vi "main.vi"() -> ()   [LabVIEW 2023]
uses:
  VoltageDataAquisition/VoltageDataAquisition.lvlib
panel:
  in  "Select Module":i32(ring)=-1 caption="Select Module\nTo send Request to" items=["All"=-1]
  in  "List":i32[](listbox)
  in  "delete":bool
  in  "add":bool
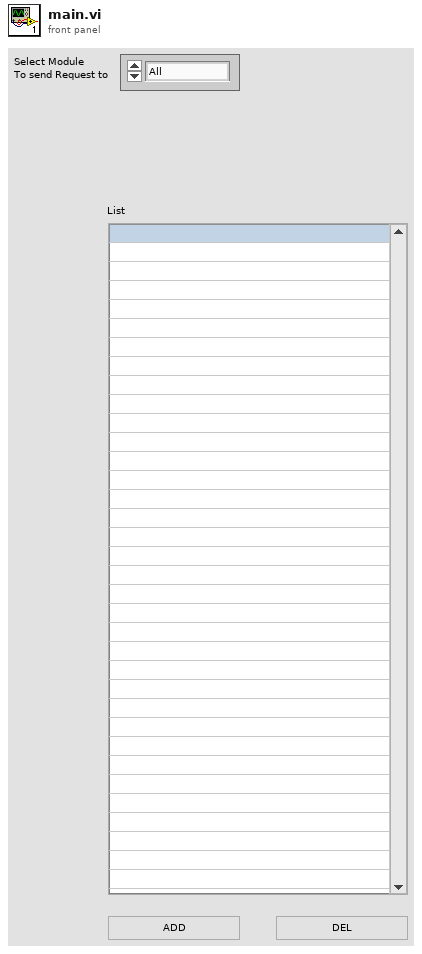
[diagram p1: front panel]
types:
  T1 = typedef "VoltageDataAquisition.lvlib/Broadcast Events--cluster.ctl" = cluster{"Module Did Init":refnum<user-event>, "Status Updated":refnum<user-event>, "Error Reported":refnum<user-event>, "Module Did Stop":refnum<user-event>, "Update Module Execution Status":refnum<user-event>}
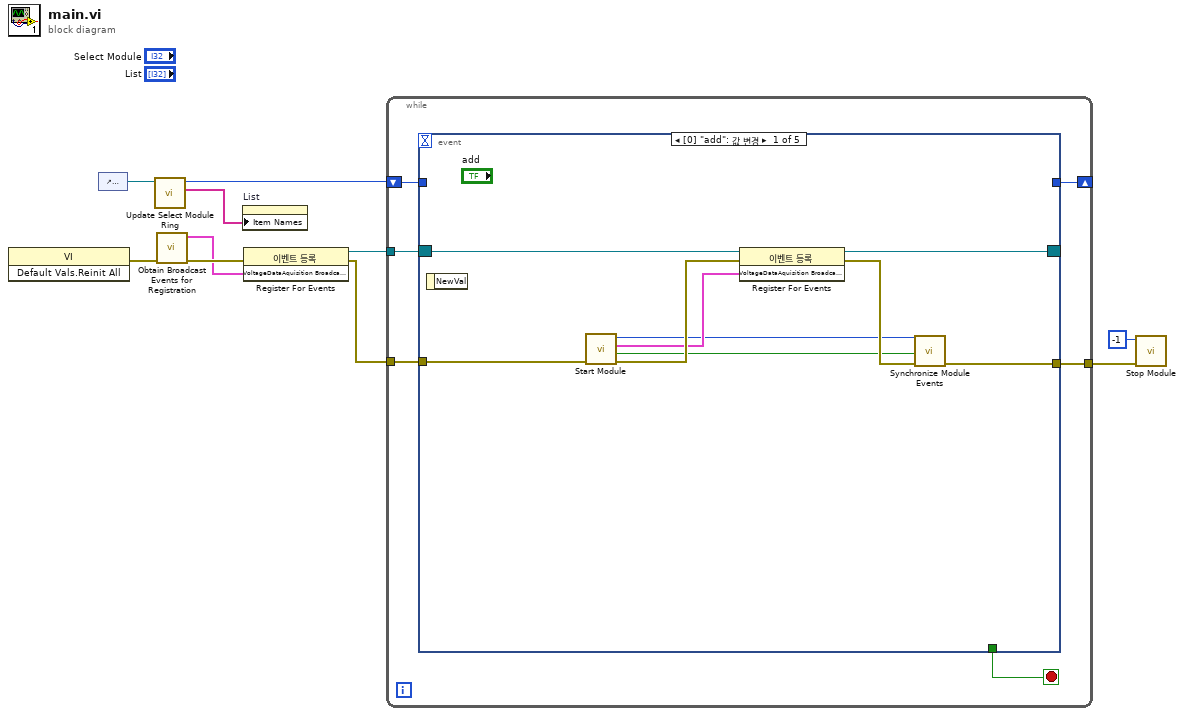
[diagram p0: block diagram]
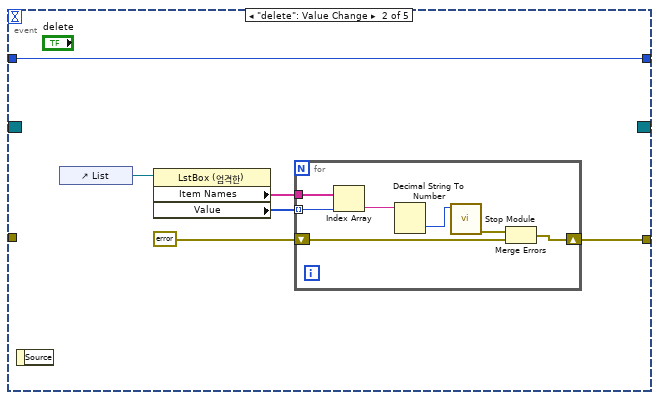
[diagram p2: hidden frame]
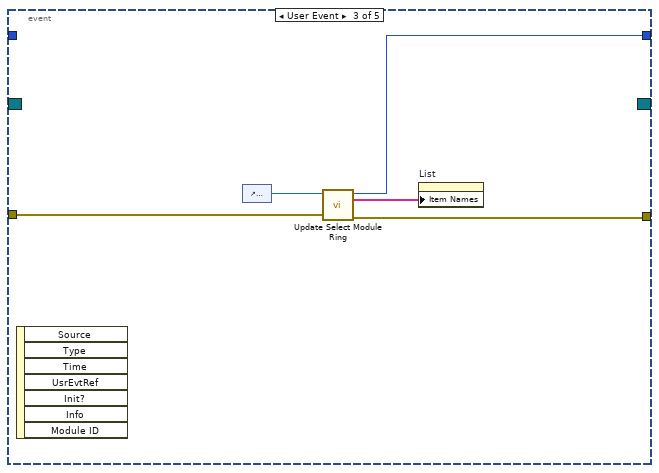
[diagram p3: hidden frame]
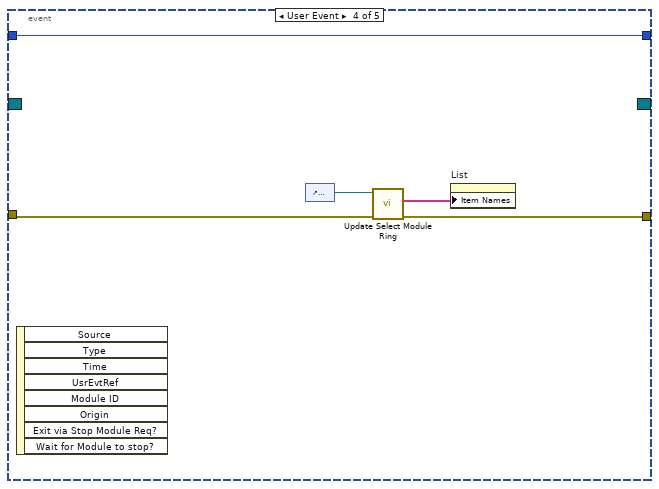
[diagram p4: hidden frame]
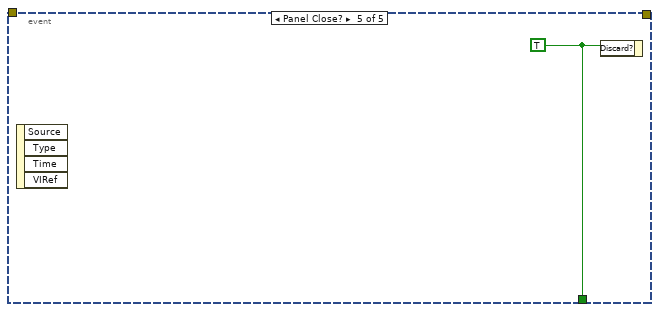
[diagram p5: hidden frame]
diagram:
  n1 = invoke class="VI" method="Default Vals.Reinit All"() -> (error out=w10:errorcluster)  [unwired: 3 in, 2 out]
  n2 = control-ref of="Select Module"() -> (w3:refnum<vi>)
  n3 = call "Update Select Module Ring.vi"("Select Module Ring Ref"=w3) -> ("Active Modules (Array)"=w1:string[], "New Module Ring Value"=w2:i32)  [unwired: 8 in, 1 out]
  n4 = call "Obtain Broadcast Events for Registration.vi"("error in"=w10) -> ("error out"=w9:errorcluster, "VoltageDataAquisition Broadcast Events"=w8:T1)  [unwired: 8 in, 1 out]
  n5 = property on="List" class="LstBox (엄격한)"("Item Names"=w1) -> ()  [unwired: 2 in, 2 out]
  n6 = register-events(error in=w9, w8) -> (reference out=w7:refnum<event-registration>, error out=w6:errorcluster)  [unwired: 1 in]
  n7 = while {
    tunnel: w7 -> [w16]
    tunnel: w6 -> [w15]
    tunnel: [w13] -> w4
    shift-right: [w11] -> _
    shift-left: w2 -> [w12]
    stop <- w14 stop-if-true
    n8 = event shown="[0] \"add\": 값 변경" {
      selector: w16 -> [w23 _ _ _ _]
      dyn-events: [w20 _ _ _ _] -> _
      timeout: _ -> [_ _ _ _ _]
      tunnel: w15 -> [w22 _ w43 w45 _]
      tunnel: [w18 w28 w42 w48 _] -> w13
      tunnel: [_ _ _ _ w49] -> w14
      tunnel: w12 -> [_ w26 _ w47 _]
      tunnel: [_ w26 w39 w47 _] -> w11
      event "add": Value Change {
        n9 = event-data() -> ()  [unwired: 1 in, 1 out]
        n10 = call "Start Module.vi"("error in"=w22) -> ("error out"=w25:errorcluster, "Wait for Event Sync?"=w17:bool, "VoltageDataAquisition Broadcast Events"=w24:T1, "Module ID"=w19:i32)  [unwired: 7 in]
        n11 = register-events(reference=w23, error in=w25, w24) -> (reference out=w20:refnum<event-registration>, error out=w21:errorcluster)
        n12 = call "Synchronize Module Events.vi"("error in"=w21, "Wait for Event Sync?"=w17, "Module ID in"=w19) -> ("error out"=w18:errorcluster)  [unwired: 7 in, 1 out]
      }
      event "delete": Value Change {
        n13 = event-data() -> ()  [unwired: 1 in, 1 out]
        n14 = control-ref of="List"() -> (w31:refnum<vi>)
        n15 = property class="LstBox (엄격한)"(reference=w31) -> ("Item Names"=w30:string[], "Value"=w29:i32[])  [unwired: 1 in, 2 out]
        n16 = for {
          tunnel: w30 -> [w38]
          tunnel: w29 -> [w37] mode=indexing
          shift-right: [w34] -> w28
          shift-left: errorcluster {"status"=FALSE, "code"=0, "source"=""} ("에러 상수") -> [w33]
          n17 = Index Array(array=w38, index=w37) -> (element=w36:string)
          n18 = Decimal String To Number(string=w36) -> (number=w32:i32)  [unwired: 2 in, 1 out]
          n19 = call "Stop Module.vi"("Module ID"=w32) -> ("error out"=w35:errorcluster)  [unwired: 10 in]
          n20 = Merge Errors(w35, w33) -> (w34:errorcluster)
        }
      }
      event User Event {
        n21 = event-data() -> ()  [unwired: 1 in, 7 out]
        n22 = control-ref of="Select Module"() -> (w40:refnum<vi>)
        n23 = call "Update Select Module Ring.vi"("error in"=w43, "Select Module Ring Ref"=w40) -> ("error out"=w42:errorcluster, "Active Modules (Array)"=w41:string[], "New Module Ring Value"=w39:i32)  [unwired: 7 in]
        n24 = property on="List" class="LstBox (엄격한)"("Item Names"=w41) -> ()  [unwired: 2 in, 2 out]
      }
      event User Event {
        n25 = event-data() -> ()  [unwired: 1 in, 8 out]
        n26 = control-ref of="Select Module"() -> (w46:refnum<vi>)
        n27 = call "Update Select Module Ring.vi"("error in"=w45, "Select Module Ring Ref"=w46) -> ("error out"=w48:errorcluster, "Active Modules (Array)"=w44:string[])  [unwired: 7 in, 1 out]
        n28 = property on="List" class="LstBox (엄격한)"("Item Names"=w44) -> ()  [unwired: 2 in, 2 out]
      }
      event Panel Close? {
        w49 = TRUE
        n29 = event-data() -> ()  [unwired: 1 in, 4 out]
        n30 = event-data("Discard?"=w49) -> ()  [unwired: 1 in, 1 out]
      }
    }
  }
  n31 = call "Stop Module.vi"("error in"=w4, "Module ID"=-1) -> ()  [unwired: 9 in, 1 out]
